vi "z closure sample call.vi"(8 "error in (no error)":errorcluster, 10 "sample":cluster{}, 11 "closure":cluster{}) -> (0 "error out":errorcluster, 2 "sample out":cluster{})   [LabVIEW 2021, in "zenohc.lvlib"]
doc: "void z_closure_sample_call(const struct z_loaned_closure_sample_t *closure,\n struct z_loaned_sample_t *sample);"
uses:
  zenohc.lvlib
  zenohc.dll
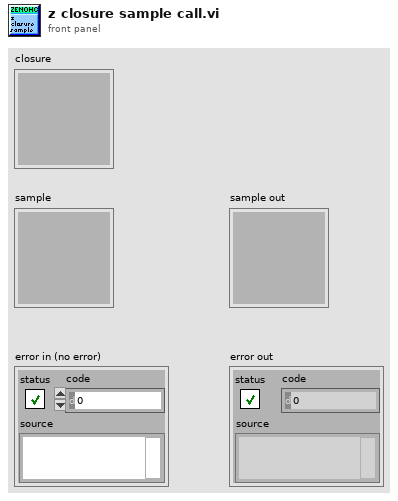
[diagram p1: front panel]
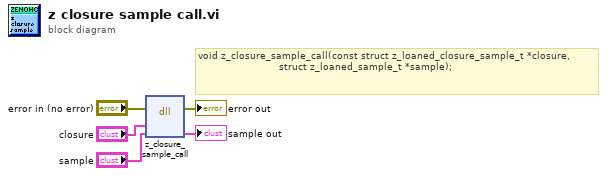
[diagram p0: block diagram]
diagram:
  # "void z_closure_sample_call(const struct z_loaned_closure_sample_t *closure,\n                           struct z_loaned_sample_t *sample);"
  n1 = dll-call lib="D:/dev/zenoh_labview/zenohc/zenohc.*" fn="z_closure_sample_call"(error in="error in (no error)", "closure"="closure", "sample"="sample") -> (error out=→"error out":errorcluster, "sample"=→"sample out":cluster{})  [unwired: 4 in, 1 out]
